vi "Get Parameter Value - core.vi"(8 "error in (no error)":errorcluster, 9 "Parameter name":string, 10 "Config name":string, 11 "Config in":refnum<class "Config.lvclass">) -> (0 "error out":errorcluster, 2 "Value":string, 3 "Config out":refnum<class "Config.lvclass">)   [LabVIEW 2026, in "TALOS.lvlib" / "Classes.lvlib" / "Config.lvclass"]
uses:
  Config.lvclass
  Config.lvclass/Config.ctl
  TALOS.lvlib
panel:
  in  "Default value":string
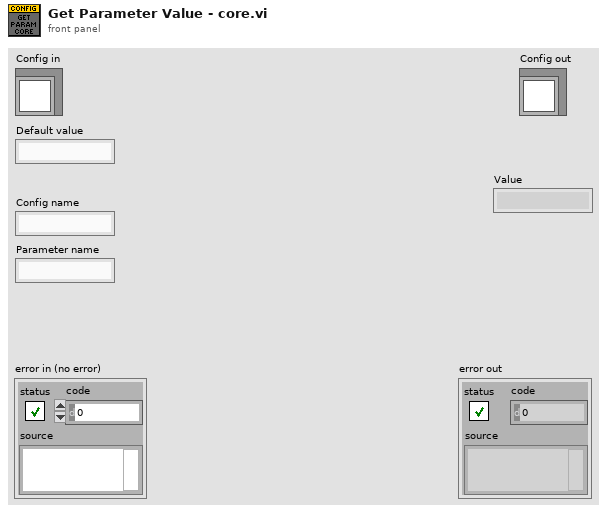
[diagram p1: front panel]
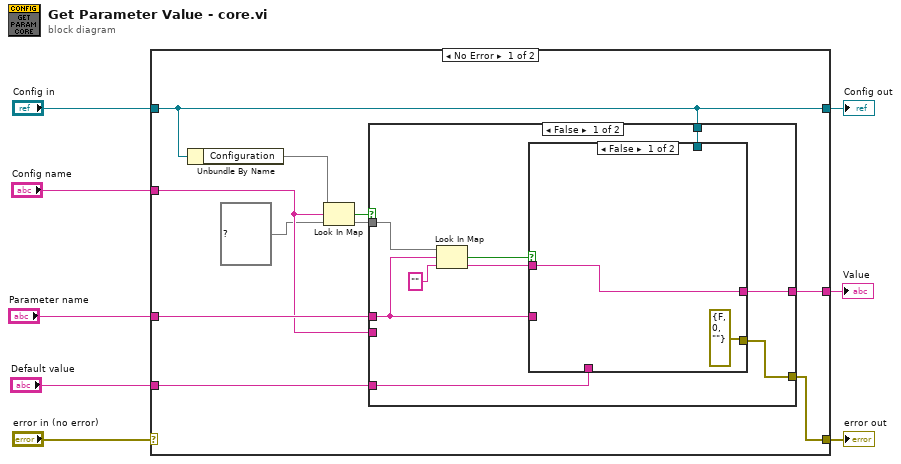
[diagram p0: block diagram]
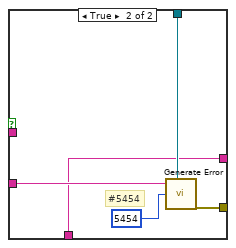
[diagram p2: hidden frame]
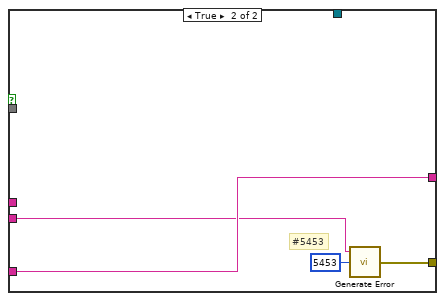
[diagram p3: hidden frame]
diagram:
  n1 = case shown="No Error" "error in (no error)" {
    selector: "error in (no error)" -> [_ w41]
    tunnel: [w15 w41] -> w1
    tunnel: [w12 w40] -> w3
    tunnel: "Config in" -> [w12 w40]
    tunnel: "Parameter name" -> [w16 _]
    tunnel: [w13 w39] -> w2
    tunnel: "Default value" -> [w11 w39]
    tunnel: "Config name" -> [w10 _]
    frame No Error {
      n2 = Unbundle By Name(w12) -> ("Configuration"=w18:map{string, map{string, string}})
      n3 = Look In Map(map=w18, key=w10, default value=map{string, string} {}) -> (key not found?=w14:bool, value=w17:map{string, string})
      n4 = case shown="False" w14 {
        tunnel: w10 -> [_ w35]
        tunnel: w17 -> [w23 _]
        tunnel: w16 -> [w22 _]
        tunnel: [w25 w37] -> w15
        tunnel: [w27 w36] -> w13
        tunnel: w12 -> [w26 _]
        tunnel: w11 -> [w24 w36]
        frame False {
          n5 = Look In Map(map=w23, key=w22, default value="") -> (key not found?=w20:bool, value=w19:string)
          n6 = case shown="False" w20 {
            tunnel: w19 -> [w29 _]
            tunnel: [w29 w30] -> w27
            tunnel: w26 -> [_ w33]
            tunnel: [errorcluster {"status"=FALSE, "code"=0, "source"=""} ("error out") w34] -> w25
            tunnel: w22 -> [_ w32]
            tunnel: w24 -> [_ w30]
            frame False {
            }
            frame True {
              # "#5454"
              n7 = call "Generate Error.vi"("Optional String"=w32, "Class"=w33, "Error Code"=5454) -> ("error out"=w34:errorcluster)  [unwired: 4 in]
            }
          }
        }
        frame True {
          # "#5453"
          n8 = call "Generate Error.vi"("Optional String"=w35, "Error Code"=5453) -> ("error out"=w37:errorcluster)  [unwired: 5 in]
        }
      }
    }
    frame Error {
    }
  }
  "error out" <- w1
  "Config out" <- w3
  "Value" <- w2
